vi "Test Create a Logger with TDMS Sink as Default Config.vi"(11 "Test Case In":refnum<class "TDMS Sink.lvclass">) -> (0 "error out":errorcluster, 3 "Test Case Out":refnum<class "TDMS Sink.lvclass">)   [LabVIEW 2020, in "TDMS Sink.lvclass"]
uses:
  TDMS Sink.lvclass
  C:/Program Files (x86)/National Instruments/LabVIEW 2020/vi.lib/Astemes/LUnit/Test Case.lvclass
  Source/Type Defs/Debug Level.ctl
  <vilib>/Astemes/LUnit/Test Case.lvclass/Test Case.ctl
  167adff6-126f-4cd3-a0fe-fb5614c91eea.vi
  57feee8f-6a0f-4aca-a361-c78af3fc4574.vi
  83aa5640-88af-4d40-897c-a658cddb0844.vi
  <vilib>/Astemes/LUnit/Core/LUnit Test Case/Private/Append Fail Result.vi
  <vilib>/Astemes/LUnit/Core/LUnit Test Case/Private/Append Pass Result.vi
  167adff6-126f-4cd3-a0fe-fb5614c91eea.vi/9c5d11cd-9439-4240-a1ee-d9baace9c924.vi
  57feee8f-6a0f-4aca-a361-c78af3fc4574.vi/9c5d11cd-9439-4240-a1ee-d9baace9c924.vi
  83aa5640-88af-4d40-897c-a658cddb0844.vi/9c5d11cd-9439-4240-a1ee-d9baace9c924.vi
  <vilib>/Astemes/LUnit/Core/LUnit Test Case/Private/Run In UI.vi
  <vilib>/Utility/error.llb/Clear Errors.vi
  Source/Sinks/TDMS Sink/TDMS Sink.lvclass
  C:/Users/hughe_cx/Documents/05_repos/LVLog/Source/Sinks/Sink/Sink.lvclass
  TDMS Sink.lvclass/TDMS Sink.ctl
  Source/LV Log.lvlib
  Source/Logger/Logger.lvclass
  <vilib>/Astemes/LUnit/Test Case.lvclass
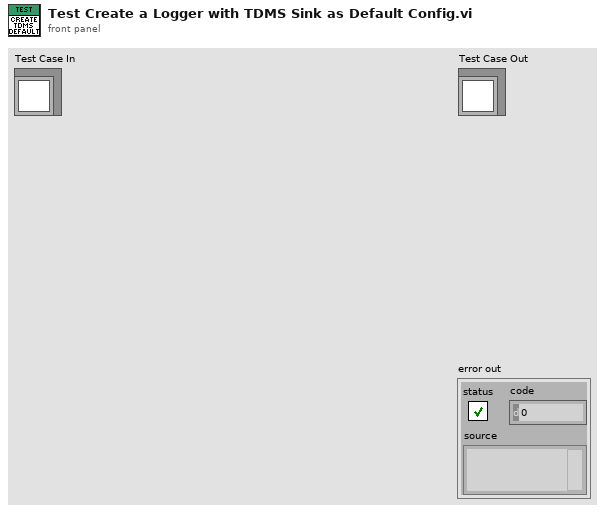
[diagram p1: front panel]
types:
  T1 = typedef "LV Log.lvlib/Debug Level.ctl" = enum16{"DEFAULT", "DEBUG", "INFO", "WARN", "ERROR", "FATAL"}
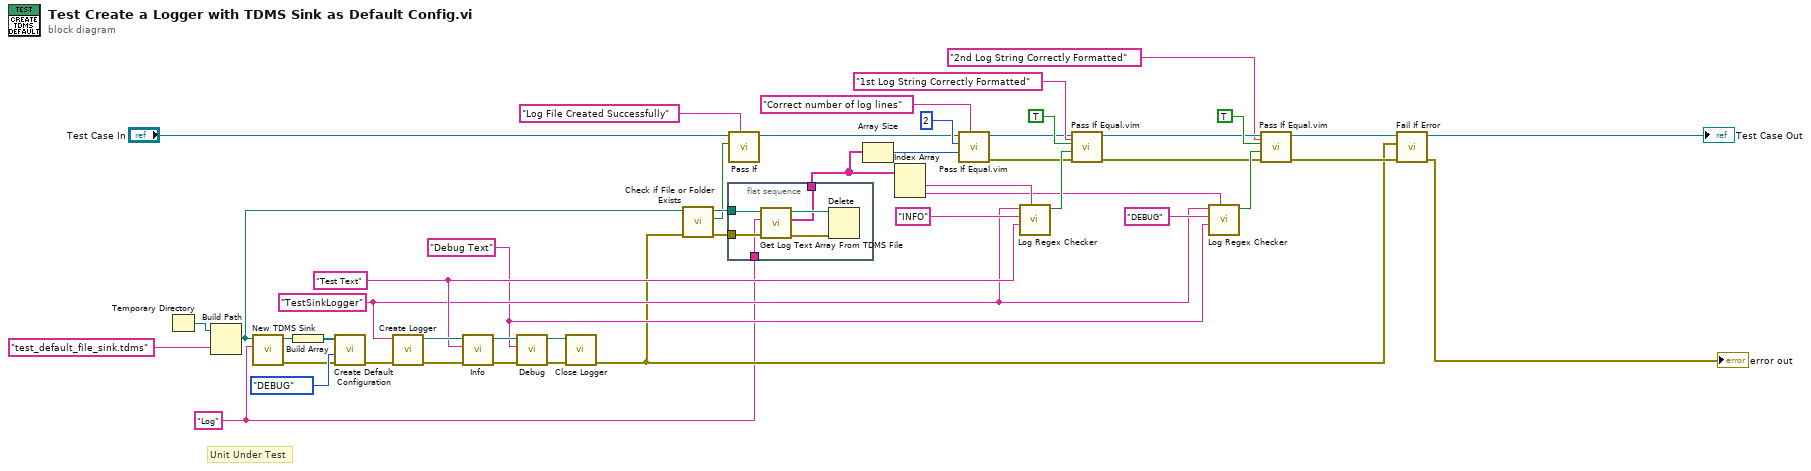
[diagram p0: block diagram]
diagram:
  w6 = "Log" ("Group Name")
  w30 = "Debug Text" ("Log Text")
  w39 = "Test Text" ("Log Text")
  w31 = "TestSinkLogger" ("Name")
  # "Unit Under Test"
  n1 = Temporary Directory() -> (w45:path)
  n2 = Build Path(base path=w45, name or relative path="test_default_file_sink.tdms" ("format string")) -> (appended path=w7:path)
  n3 = call "New TDMS Sink.vi"("Group Name"=w6, "TDMS File Path"=w7) -> ("error out"=w9:errorcluster, "TDMS out"=w8:refnum<class "TDMS Sink.lvclass">)  [unwired: 8 in]
  n4 = Build Array(w8) -> (w46:refnum<class "TDMS Sink.lvclass">[])
  n5 = call "Create Default Configuration.vi"("Sinks"=w46, "Debug Level in"=Debug_Level."DEBUG", "error in (no error)"=w9) -> ("error out"=w47:errorcluster)  [unwired: 7 in]
  n6 = call "Create Logger.vi"("error in (no error)"=w47, "Name"=w31) -> ("error out"=w43:errorcluster, "Logger out"=w42:refnum<class "Logger.lvclass">)  [unwired: 8 in]
  n7 = call "Info.vi"("error in (no error)"=w43, "Log Text"=w39, "Logger in"=w42) -> ("error out"=w38:errorcluster, "Logger out"=w37:refnum<class "Logger.lvclass">)  [unwired: 6 in, 1 out]
  n8 = call "Debug.vi"("error in (no error)"=w38, "Log Text"=w30, "Logger in"=w37) -> ("error out"=w12:errorcluster, "Logger out"=w11:refnum<class "Logger.lvclass">)  [unwired: 6 in, 1 out]
  n9 = call "Close Logger.vi"("error in (no error)"=w12, "Logger in"=w11) -> ("error out"=w10:errorcluster)  [unwired: 9 in]
  n10 = call <vilib>:"Check if File or Folder Exists.vi"("error in (no error)"=w10, "path"=w7) -> ("error out"=w16:errorcluster, "file or folder exists?"=w14:bool, "dup path"=w17:path)  [unwired: 7 in]
  n11 = flat-sequence {
    tunnel: w17 -> [w52]
    tunnel: [w49] -> w24
    tunnel: w16 -> [w53]
    tunnel: w6 -> [w48]
    frame #0 {
      n12 = call "Get Log Text Array From TDMS File.vi"("error in"=w53, "Group Name"=w48, "Log File Path in"=w52) -> ("error out"=w50:errorcluster, "Log Text Array"=w49:string[], "Log File Path out"=w51:path)  [unwired: 6 in]
      n13 = Delete(path (use dialog)=w51, error in=w50) -> ()  [unwired: 3 in, 3 out]
    }
  }
  n14 = call <vilib>:"Pass If.vi"("Description"="Log File Created Successfully", "Pass?"=w14, "LUnit Test Case In"="Test Case In") -> ("LUnit Test Case Out"=w15:refnum<class "TDMS Sink.lvclass">)  [unwired: 7 in, 1 out]
  n15 = Array Size(array=w24) -> (size(s)=w23:i32)
  n16 = Index Array(array=w24) -> (element #1=w29:string, element #2=w28:string)  [unwired: 2 in]
  n17 = call "Pass If Equal.vim"("Description"="Correct number of log lines", "Actual"=w23, "Expected"=2, "LUnit Test Case In"=w15) -> ("error out"=w18:errorcluster, "LUnit Test Case Out"=w25:refnum<class "TDMS Sink.lvclass">)  [unwired: 6 in]
  n18 = call "Log Regex Checker.vi"("Log String"=w29, "Expected Log Text (Any)"=w39, "Expected Log Level (Any)"="INFO", "Expected Logger Name (Any)"=w31) -> ("Math Found"=w35:bool)  [unwired: 5 in, 2 out]
  n19 = call "Pass If Equal.vim"("Description"="1st Log String Correctly Formatted", "error in (no error)"=w18, "Actual"=w35, "Expected"=TRUE, "LUnit Test Case In"=w25) -> ("error out"=w19:errorcluster, "LUnit Test Case Out"=w27:refnum<class "TDMS Sink.lvclass">)  [unwired: 5 in]
  n20 = call "Log Regex Checker.vi"("Log String"=w28, "Expected Log Text (Any)"=w30, "Expected Log Level (Any)"="DEBUG", "Expected Logger Name (Any)"=w31) -> ("Math Found"=w34:bool)  [unwired: 5 in, 2 out]
  n21 = call "Pass If Equal.vim"("Description"="2nd Log String Correctly Formatted", "error in (no error)"=w19, "Actual"=w34, "Expected"=TRUE, "LUnit Test Case In"=w27) -> ("error out"=w20:errorcluster, "LUnit Test Case Out"=w26:refnum<class "TDMS Sink.lvclass">)  [unwired: 5 in]
  n22 = call <vilib>:"Fail If Error.vi"("error in (no error)"=w20, "Assert error"=w10, "LUnit Test Case In"=w26) -> ("error out"=→"error out":errorcluster, "LUnit Test Case Out"=→"Test Case Out":refnum<class "TDMS Sink.lvclass">)  [unwired: 7 in]
